vi "Configure.vi"(8 "error in (no error)":errorcluster, 11 "Stage_MadCityLabMicro in":refnum<class "Stage_MadCityLabMicro.lvclass">) -> (0 "error out":errorcluster, 3 "Stage_MadCityLabMicro out":refnum<class "Stage_MadCityLabMicro.lvclass">)   [LabVIEW 2020, in "Stage_MadCityLabMicro.lvlib" / "Stage_MadCityLabMicro.lvclass"]
uses:
  Stage_MadCityLabMicro.lvclass
  Hardware Abstraction Layer/Component/Device/Device/DataExchange.ctl
  Hardware Abstraction Layer/Component/Stage/Stage/Stage.lvclass
  Interface/DataListener/DataListener.lvclass
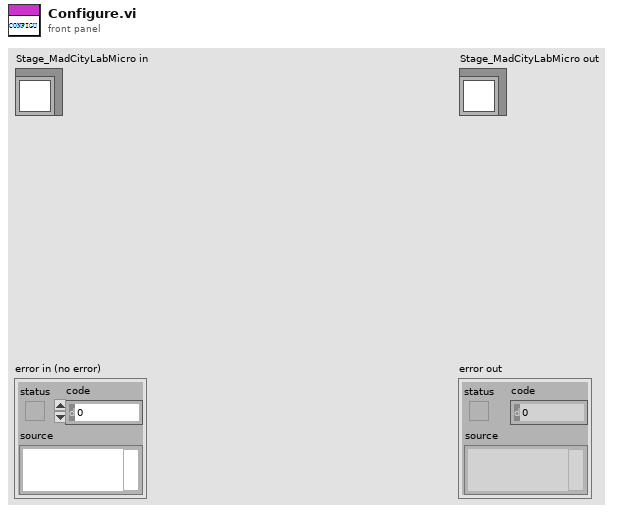
[diagram p1: front panel]
types:
  T1 = typedef "DataListener.lvclass/DataExchange.ctl" = cluster{"Source":string, "Destination":string, "Description":string, "value":variant}
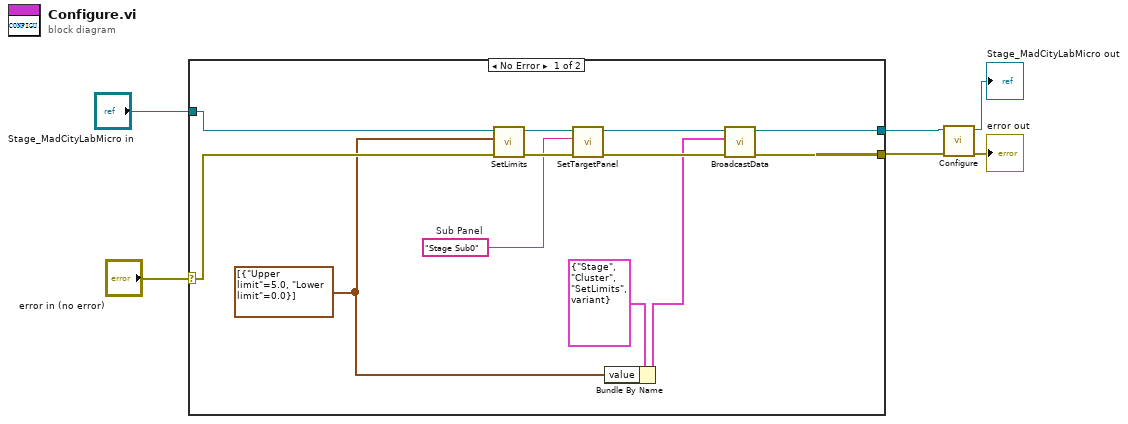
[diagram p0: block diagram]
diagram:
  n1 = case shown="No Error" "error in (no error)" {
    selector: "error in (no error)" -> [w17 w20]
    tunnel: [w12 w20] -> w1
    tunnel: [w10 w19] -> w2
    tunnel: "Stage_MadCityLabMicro in" -> [w18 w19]
    frame No Error {
      w13 = "Stage Sub0"  # Sub Panel
      w7 = cluster{"Upper limit":dbl, "Lower limit":dbl}[] [{"Upper limit"=5.0, "Lower limit"=0.0}] ("Limits")
      n2 = call-dynamic "SetLimits.vi"("error in (no error)"=w17, "Limits"=w7, "Stage in"=w18) -> ("error out"=w16:errorcluster, "Stage out"=w14:refnum<class "Stage_MadCityLabMicro.lvclass">)  [unwired: 7 in]
      n3 = call-dynamic "SetTargetPanel.vi"("error in (no error)"=w16, "TargetPanel"=w13, "GRMActor in"=w14) -> ("error out"=w15:errorcluster, "GRMActor out"=w11:refnum<class "Stage_MadCityLabMicro.lvclass">)  [unwired: 7 in]
      n4 = Bundle By Name(cluster=T1 {"Source"="Stage", "Destination"="Cluster", "Description"="SetLimits", "value"=variant} ("DataExchange"), "value"=w7) -> (w8:T1)
      n5 = call-dynamic "BroadcastData.vi"("error in (no error)"=w15, "DataExchange"=w8, "GRMActor in"=w11) -> ("error out"=w12:errorcluster, "GRMActor out"=w10:refnum<class "Stage_MadCityLabMicro.lvclass">)  [unwired: 7 in]
    }
    frame Error {
    }
  }
  n6 = call-parent "Configure.vi"("error in (no error)"=w1, "Device in"=w2) -> ("error out"=→"error out":errorcluster, "Device out"=→"Stage_MadCityLabMicro out":refnum<class "Stage_MadCityLabMicro.lvclass">)  [unwired: 8 in]
